vi "SPI.Get Bob ID.vi"() -> (3 "Bob.ID":u8=5)   [LabVIEW 2018]
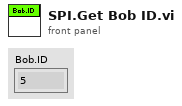
[diagram p1: front panel]
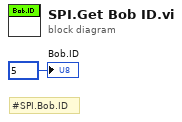
[diagram p0: block diagram]
diagram:
  # "#SPI.Bob.ID"
  "Bob.ID" <- u8 5
